vi "PH_GetCamInformation.get and prepare Info.vi"(5 "error in":errorcluster) -> (14 "Rows with conflicts":i32[](array[numeric]), 15 "ColHdrs[]":string[](array[string])=["Sixpack Instance", "Axis"], 16 "RowHdrs[]":string[](array[string]), 17 "ItemNames":string[][](array[string]), 18 "Row Cell BG":u32[](array[numeric]), 19 "error out":errorcluster)   [LabVIEW 2014, in "PH_GetCamInformation.lvlib"]
doc: "This VI is reading out information from the database and prepares it for the visualisation on the GUI."
uses:
  PH_GetCamInformation.lvlib
  PH_Common/PH_Common.lvlib
  CSCore/CSSystem/CSSystemLib/CSSystemLib.lvlib
  PH_Cam_BaseClass/PH_Cam_BaseClass.lvlib
  lib.lib/DimLVEvent/LVDimInterface/LVDimInterface.lvlib
  CSCore/CSSystem/CoreLib/CoreLib.lvlib
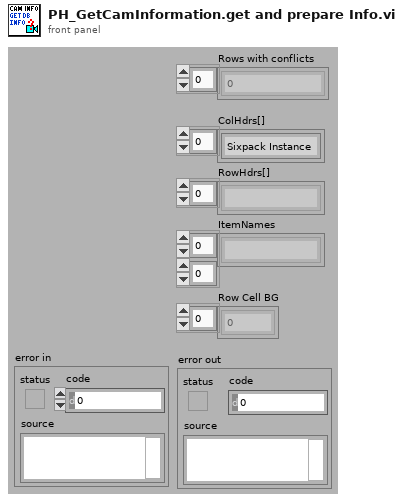
[diagram p1: front panel]
types:
  T1 = typedef "PH_Cam_BaseClass.lvlib/PH_Cam_BaseClass.Settings.ctl" = cluster{"Cam ID":string, "Gain":dbl, "Brightness":dbl, "Shutter":dbl, "Mode":i32}
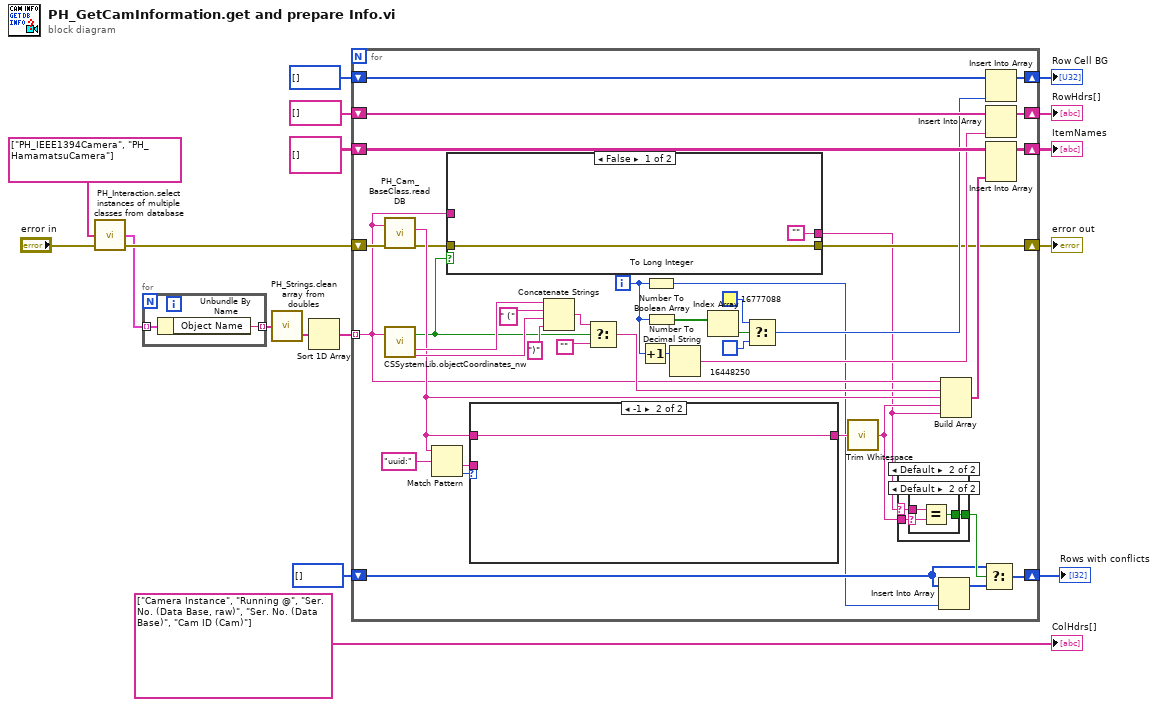
[diagram p0: block diagram]
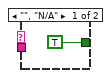
[diagram p2: hidden frame]
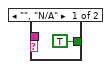
[diagram p3: hidden frame]
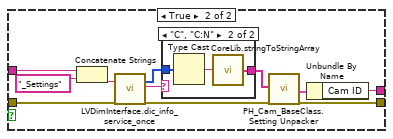
[diagram p4: hidden frame]
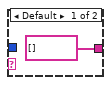
[diagram p5: hidden frame]
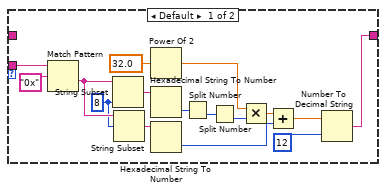
[diagram p6: hidden frame]
diagram:
  n1 = call "PH_Interaction.select instances of multiple classes from database.vi"("error in (no error)"="error in", "Classes Input"=string[] ["PH_IEEE1394Camera", "PH_HamamatsuCamera"]) -> ("error out"=w10:errorcluster, "Query Result"=w9:cluster{"Object Name":string, "Class":string}[])  [unwired: 2 in]
  n2 = for {
    tunnel: w9 -> [w19] mode=indexing
    tunnel: [w18] -> w8 mode=indexing
    n3 = Unbundle By Name(w19) -> ("Object Name"=w18:string)
  }
  n4 = call "PH_Strings.clean array from doubles.vi"("Array Input"=w8) -> ("Cleaned Array Output"=w7:string[])  [unwired: 1 out]
  n5 = Sort 1D Array(array=w7) -> (sorted array=w6:string[])
  n6 = for {
    tunnel: w6 -> [w30] mode=indexing
    shift-right: [w58] -> w3
    shift-left: string[][] [] -> [w57]
    shift-right: [w54] -> w15
    shift-left: string[] [] -> [w55]
    shift-right: [w52] -> w17
    shift-left: u32[] [] -> [w51]
    shift-right: [w31] -> w4
    shift-left: w10 -> [w33]
    shift-right: [w26] -> w1
    shift-left: i32[] [] -> [w24]
    i -> [w23]
    n7 = call "PH_Cam_BaseClass.read DB.vi"("DB Entry to read"=w30, "error in (no error)"=w33) -> ("Camera ID"=w34:string, "error out"=w32:errorcluster)  [unwired: 2 out]
    n8 = call "CSSystemLib.objectCoordinates_nw.vi"("name"=w30) -> ("obj exists"=w29:bool, "systemID"=w48:string, "node"=w45:string)  [unwired: 15 in, 1 out]
    n9 = Match Pattern(string=w34, regular expression="uuid:") -> (after substring=w35:string, offset past match=w36:i32)  [unwired: 1 in, 2 out]
    n10 = case shown="False" w29 {
      tunnel: w32 -> [w68 w75]
      tunnel: [w68 w73] -> w31
      tunnel: w30 -> [_ w70]
      tunnel: ["" w69] -> w20
      frame False {
      }
      frame True {
        n11 = Concatenate Strings(w70, "_Settings" ("string")) -> (w71:string)
        n12 = call "LVDimInterface.dic_info_service_once.vi"("serviceName"=w71, "error in (no error)"=w75) -> ("data"=w77:i8[], "typeDescriptor"=w78:string, "error out"=w74:errorcluster)  [unwired: 14 in, 1 out]
        n13 = case shown="\"C\", \"C:N\"" w78 {
          tunnel: w77 -> [_ w83]
          tunnel: [string[] [] ("Array") w81] -> w76
          frame Default {
          }
          frame "C", "C:N" {
            n14 = Type Cast(x=w83) -> (*(type *) &x=w82:string)  [unwired: 1 in]
            n15 = call "CoreLib.stringToStringArray.vi"("String"=w82) -> ("Array"=w81:string[])
          }
        }
        n16 = call "PH_Cam_BaseClass.Setting Unpacker.vi"("Cam Settings Array"=w76, "error in (no error)"=w74) -> ("Cam Settings"=w79:T1, "error out"=w73:errorcluster)  [unwired: 15 in, 1 out]
        n17 = Unbundle By Name(w79) -> ("Cam ID"=w69:string)
      }
    }
    n18 = case shown="-1" w36 {
      tunnel: [w85 w100] -> w28
      tunnel: w34 -> [_ w100]
      tunnel: w35 -> [w98 _]
      frame Default {
        w96 = 8 ("length (rest)")
        n19 = Match Pattern(string=w98, regular expression="0x") -> (after substring=w97:string)  [unwired: 1 in, 3 out]
        n20 = String Subset(string=w97, length (rest)=w96) -> (substring=w90:string)  [unwired: 1 in]
        n21 = String Subset(string=w97, offset (0)=w96) -> (substring=w89:string)  [unwired: 1 in]
        n22 = Power Of 2(x=32.0) -> (2^x=w94:dbl)
        n23 = Hexadecimal String To Number(string=w90) -> (number=w88:u32)  [unwired: 2 in, 1 out]
        n24 = Hexadecimal String To Number(string=w89) -> (number=w87:u32)  [unwired: 2 in, 1 out]
        n25 = Split Number(x=w88) -> (lo(x)=w92:u16)  [unwired: 1 out]
        n26 = Split Number(x=w92) -> (lo(x)=w91:u8)  [unwired: 1 out]
        n27 = Multiply(x=w94, y=w91) -> (x*y=w93:dbl)
        n28 = Add(x=w93, y=w87) -> (x+y=w84:dbl)
        n29 = Number To Decimal String(number=w84, width (-)=i16 12) -> (decimal integer string=w85:string)
      }
      frame -1 {
      }
    }
    n30 = Concatenate Strings(w48, " (" ("string"), w45, ")" ("string")) -> (w47:string)
    n31 = Select(t=w47, s=w29, f="") -> (s? t:f=w49:string)
    n32 = Increment(x=w23) -> (x+1=w42:i32)
    n33 = To Long Integer(number=w23) -> (32bit integer=w22:i32)
    n34 = Number To Boolean Array(number=w23) -> (Boolean array=w40:bool[])
    n35 = Number To Decimal String(number=w42) -> (decimal integer string=w56:string)  [unwired: 1 in]
    n36 = Index Array(array=w40) -> (element=w41:bool)  [unwired: 1 in]
    n37 = Select(t=u32 16777088 ("Color Box"), s=w41, f=u32 16448250 ("Color Box")) -> (s? t:f=w53:u32)
    n38 = call <vilib>:"Trim Whitespace.vi"("string"=w28) -> ("trimmed string"=w21:string)  [unwired: 1 in]
    n39 = case shown="Default" w20 {
      selector: w20 -> [_ w60]
      tunnel: [TRUE w62] -> w27
      tunnel: w21 -> [_ w61]
      frame "", "N/A" {
      }
      frame Default {
        n40 = case shown="Default" w61 {
          selector: w61 -> [_ w64]
          tunnel: w60 -> [_ w66]
          tunnel: [TRUE w65] -> w62
          frame "", "N/A" {
          }
          frame Default {
            n41 = Equal?(x=w66, y=w64) -> (x = y?=w65:bool)
          }
        }
      }
    }
    n42 = Insert Into Array(array=w24, new element=w22) -> (w25:i32[])  [unwired: 1 in]
    n43 = Build Array(w30, w49, w34, w21, w20) -> (w43:string[])
    n44 = Select(t=w24, s=w27, f=w25) -> (s? t:f=w26:i32[])
    n45 = Insert Into Array(array=w51, new element=w53) -> (w52:u32[])  [unwired: 1 in]
    n46 = Insert Into Array(array=w55, new element=w56) -> (w54:string[])  [unwired: 1 in]
    n47 = Insert Into Array(array=w57, new element=w43) -> (w58:string[][])  [unwired: 2 in]
  }
  "error out" <- w4
  "Row Cell BG" <- w17
  "RowHdrs[]" <- w15
  "ItemNames" <- w3
  "Rows with conflicts" <- w1
  "ColHdrs[]" <- string[] ["Camera Instance", "Running @", "Ser. No. (Data Base, raw)", "Ser. No. (Data Base)", "Cam ID (Cam)"] ("new element/subarray")
